vi "ValidateNum.vi"(8 "Number":i32, 9 "Column":i32, 10 "Row":i32, 11 "Board":i32[][](array[numeric])) -> (0 "Number to Search":i32, 1 "Column":i32, 2 "Row":i32, 3 "Board":i32[][](array[numeric]), 4 "Valid?":bool)   [LabVIEW 2023]
doc: "Checks if Number is possible in current cell.\n\nInputs\n- Board: Current Board Configuration\n- Row: Row of current Cell\n- Column: Column of current Cell\n- Number: Number to try out in current Cell\n\nOutputs\n- Board: Current Board Configuration\n- Row: Row of current Cell\n- Column: Column of current Cell\n- Number: Number to try out in current Cell\n- Valid?: Is TRUE if Number is valid in Cell"
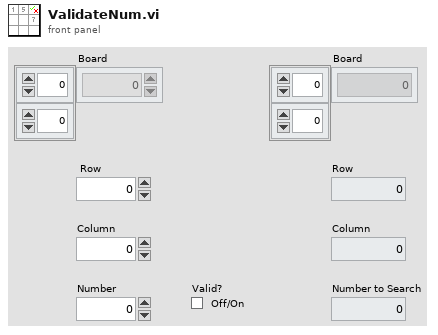
[diagram p1: front panel]
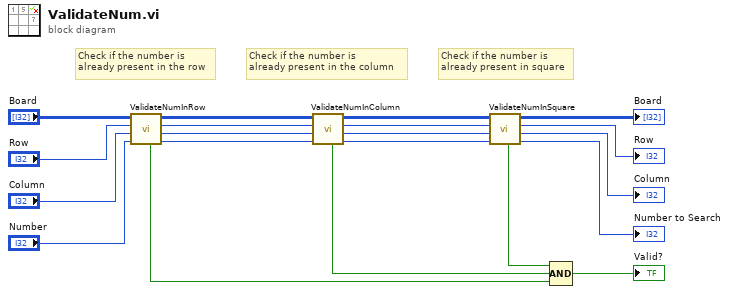
[diagram p0: block diagram]
diagram:
  # "Check if the number is \nalready present in the column"
  # "Check if the number is \nalready present in square"
  # "Check if the number is \nalready present in the row"
  n1 = call "ValidateNumInRow.vi"("Number"="Number", "Column"="Column", "Row"="Row", "Board"="Board") -> ("Number"=w7:i32, "Column"=w8:i32, "Row"=w3:i32, "Board"=w2:i32[][], "Valid in Row"=w14:bool)  [unwired: 3 in]
  n2 = call "ValidateNumInColumn.vi"("Number"=w7, "Column"=w8, "Row"=w3, "Board"=w2) -> ("Number"=w10:i32, "Column"=w9:i32, "Row"=w6:i32, "Board"=w5:i32[][], "Valid in Column"=w13:bool)  [unwired: 3 in]
  n3 = call "ValidateNumInSquare.vi"("Number"=w10, "Column"=w9, "Row"=w6, "Board"=w5) -> ("Number"=→"Number to Search":i32, "Column"=→"Column":i32, "Row"=→"Row":i32, "Board"=→"Board":i32[][], "Valid in Square"=w12:bool)  [unwired: 3 in]
  n4 = Compound Arithmetic op=AND(w12, w13, w14) -> (→"Valid?":bool)
